vi "Properties To Create.vi"(8 "error in (no error)":errorcluster, 11 "CD Template in":refnum<class "NIVS_CD Template.lvclass">) -> (0 "error out":errorcluster, 2 "Properties":T1[](array[typedef]))   [LabVIEW 2017, in "NIVS_CD Template.lvclass"]
uses:
  NIVS_CD Template.lvclass
  NIVS_Consolidated_CDW_MetaDataObj/Property Information.ctl
  NIVS_Consolidated_CDW_MetaDataObj/NIVS_Consolidated_CDW_MetaDataObj.lvclass
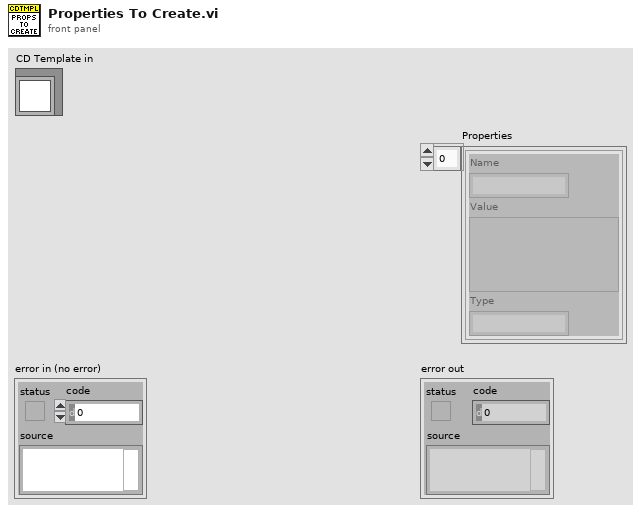
[diagram p1: front panel]
types:
  T1 = typedef "NIVS_Consolidated_CDW_MetaDataObj.lvclass/Property Information.ctl" = cluster{"Name":string, "Value":variant, "Type":string}
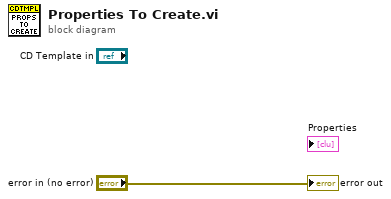
[diagram p0: block diagram]
diagram:
  "error out" <- "error in (no error)"
